vi "sub tab from criteria.vi"(1 "Criteria":T2) -> (0 "Tab Control":T1(ring)=enum."Time")   [LabVIEW 2011, in "Criteria control.xctl"]
uses:
  Criteria control.xctl
  Criteria types.ctl
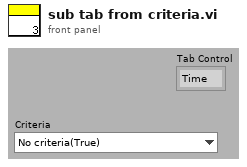
[diagram p1: front panel]
types:
  T1 = enum32{"Nothing", "One digital", "Time", "One dbl", "Two dbl"}
  T2 = typedef "Criteria types.ctl" = enum16{"No criteria(True)", "Time(s)", "Analog IO over", "Analog IO over or equal", "Analog IO under", "Analog IO under or equal", "Analog IO 1 minus Analog IO 2 over", "Digital IO True", "Digital IO False", "Operator approval"}
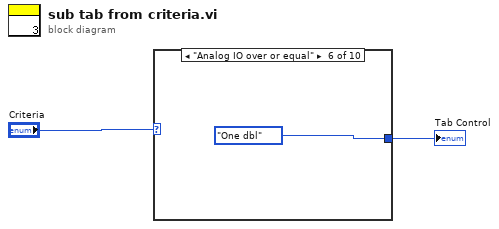
[diagram p0: block diagram]
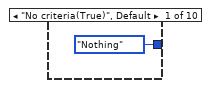
[diagram p2: hidden frame]
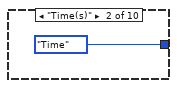
[diagram p3: hidden frame]
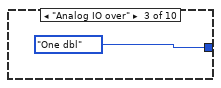
[diagram p4: hidden frame]
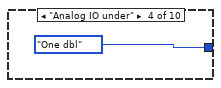
[diagram p5: hidden frame]
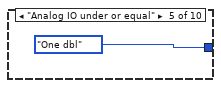
[diagram p6: hidden frame]
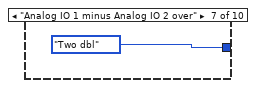
[diagram p7: hidden frame]
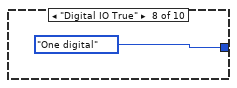
[diagram p8: hidden frame]
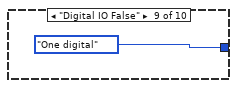
[diagram p9: hidden frame]
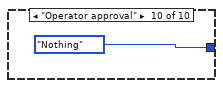
[diagram p10: hidden frame]
diagram:
  n1 = case shown="\"Analog IO over or equal\"" "Criteria" {
    tunnel: [T1."Nothing" ("Tab Control") T1."Time" ("Tab Control") T1."One dbl" ("Tab Control") T1."One dbl" ("Tab Control") T1."One dbl" ("Tab Control") T1."One dbl" ("Tab Control") T1."Two dbl" ("Tab Control") T1."One digital" ("Tab Control") T1."One digital" ("Tab Control") T1."Nothing" ("Tab Control")] -> w2
    frame "No criteria(True)", Default {
    }
    frame "Time(s)" {
    }
    frame "Analog IO over" {
    }
    frame "Analog IO under" {
    }
    frame "Analog IO under or equal" {
    }
    frame "Analog IO over or equal" {
    }
    frame "Analog IO 1 minus Analog IO 2 over" {
    }
    frame "Digital IO True" {
    }
    frame "Digital IO False" {
    }
    frame "Operator approval" {
    }
  }
  "Tab Control" <- w2
